vi "AIT 664 RT Driver VI.vi"(7 "Operation":T1, 11 "Device Reference in":T2 format="%.0x") -> (0 "Error Code":i32)   [LabVIEW 2014, in "AIT 664 Custom Device.lvlib"]
uses:
  AIT 664 Custom Device.lvlib
  <vilib>/NI Veristand/Custom Device API/Custom Device Item Ref.ctl
  <vilib>/NI Veristand/Custom Device API/Hardware Interface Driver VI Operation.ctl
  RT Controls/AIT 664  - RT Data.ctl
  RT Controls/AIT 664 - RT Hardware Channel.ctl
  RT Controls/AIT 664 - RT Message Settings.ctl
  <vilib>/NI Veristand/Custom Device API/Block Data Reference.ctl
  <vilib>/NI Veristand/Custom Device API/Data Reference.ctl
  RT Controls/AIT 664 - Driver Data.ctl
  Controls and Global/Start Bit.ctl
  Controls and Global/Number of Bits.ctl
  <userlib>/ARINC 664/AIT 664 Controls/General/Message Port.ctl
  <userlib>/ARINC 664/AIT 664 Controls/General/Direction.ctl
  <userlib>/ARINC 664/AIT 664 Controls/General/Message Port Type.ctl
  System Explorer/Controls/664 - Sampling Type.ctl
  RT Controls/Status Channels Config.ctl
  RT Controls/FIFO.ctl
  RT Controls/Label Transfer Config.ctl
  RT Controls/Async Loop Control Enum.ctl
  RT Controls/ReadWrite Selector.ctl
  SubVIs/Data Ref FGV.vi
  <vilib>/NI Veristand/Custom Device API/NI VeriStand - Set Channel Value by Data Reference.vi
  SubVIs/Error/Push Error if Different.vi
  <instrlib>/AIT 664/Private/AIT 664 Configure/Rx/Close/AIT 664 Rx Close Message Port (ComUdp).vi
  <instrlib>/AIT 664/Private/AIT 664 Configure/Tx/Close/AIT 664 Tx Close Message Port (ComUdp).vi
  <vilib>/NI Veristand/Custom Device API/Global Data Refs.vi
  SubVIs/Init/AIT 664 - Get Index and Length.vi
  SubVIs/Init/AIT 664 - Parse Channels.vi
  <vilib>/NI Veristand/Custom Device API/Custom Device API.lvlib
  <userlib>/ARINC 664/AIT 664 API.lvlib
  <instrlib>/AIT 664/AIT 664.lvlib
  <vilib>/NI Veristand/Custom Device Tools/Custom Device Utility Library/Custom Device Utility Library.lvlib
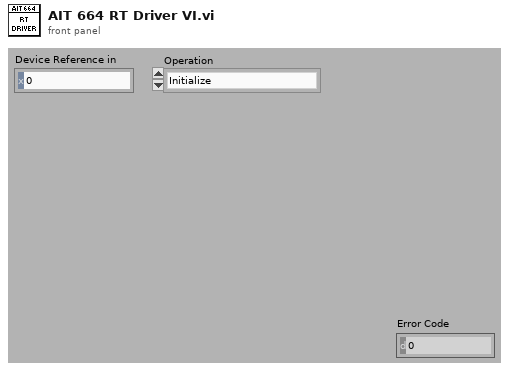
[diagram p1: front panel]
types:
  T1 = typedef "Custom Device API.lvlib/Hardware Interface Driver VI Operation.ctl" = enum16{"Initialize", "Start", "Read Data from HW", "Write Data to HW", "Close"}
  T2 = typedef "Custom Device API.lvlib/Custom Device Item Ref.ctl" = u64
  T3 = typedef "AIT 664 Custom Device.lvlib/AIT 664  - RT Data.ctl" = cluster{"Hardware Input Rx Channels":T4[], "Hardware Output Tx Channels":T4[], "Start":refnum<notifier>, "Error Publish Queue":refnum<queue>, "Error Queues":refnum<queue>[], "Status Config":T15, "FIFOs":T16, "VI References":refnum<vi>[], "Label Transfer Config":T17, "End System Handle ":u64}
  T4 = typedef "AIT 664 Custom Device.lvlib/AIT 664 - RT Hardware Channel.ctl" = cluster{"Channel Number":u16, "Message Name":string, "Message Settings":T5, "Tx Com Udp Port":T11, "Rx Com Udp Port":T11, "Rate (ms)":u32, "Sampling Type":T14}
  T5 = typedef "AIT 664 Custom Device.lvlib/AIT 664 - RT Message Settings.ctl" = cluster{"Name":string, "xmlName":string, "Tx-Rx_T-Tx":bool, "RT_Address":u8, "RT_SA_Address":u8, "Block Data Refs":T6[], "Values Array":dbl[], "Length":i32, "Words":i32, "FIFO Index":i32, "RX Word":u32, "IterationOffset":i32, "Default Msg Data":u8[], "Driver Data":T8, "Status Data":u32[], "Queue Transmit Channel":T2, "Transmit Channel Data Reference":T7}
  T6 = typedef "Custom Device API.lvlib/Block Data Reference.ctl" = cluster{"Data Reference":T7, "Offset":i32, "Length":i32}
  T7 = typedef "Custom Device API.lvlib/Data Reference.ctl" = i32
  T8 = typedef "AIT 664 Custom Device.lvlib/AIT 664 - Driver Data.ctl" = cluster{"First Word":T9[], "Start Bit":T9[], "Num Bits":T10[], "Decimation":i32, "IterationOffset":i32, "Signed?":bool[], "ScaleFac":dbl[], "ScaleOffset":dbl[]}
  T9 = typedef "AIT 664 Custom Device.lvlib/Start Bit.ctl" = i32
  T10 = typedef "AIT 664 Custom Device.lvlib/Number of Bits.ctl" = i32
  T11 = typedef "AIT 664 API.lvlib/Message Port.ctl" = cluster{"Direction":T12, "Type":T13, "Handle":u64}
  T12 = typedef "AIT 664 API.lvlib/Direction.ctl" = enum16{"DIRECTION_NONE", "DIRECTION_TX", "DIRECTION_RX"}
  T13 = typedef "AIT 664 API.lvlib/Message Port Type.ctl" = enum16{"PORT_TYPE_NONE", "COM_UDP", "SAP_UDP", "SAP_IP", "SAP_MAC", "COTS_MAC", "COTS_MAC_RAW"}
  T14 = typedef "AIT 664 Custom Device.lvlib/664 - Sampling Type.ctl" = enum16{"Com Udp", "Com Udp Queuing", "Sap Udp", "Sap Ip", "Sap Mac", "Unknown"}
  T15 = typedef "AIT 664 Custom Device.lvlib/Status Channels Config.ctl" = cluster{"Error Data Reference":T7, "Hardware In Count Reference":T7, "Hardware In Count Index":i32, "Hardware Out Count Reference":T7, "Hardware Out Count Index":i32, "Hardware In Dur Reference":T7, "Hardware In Dur Index":i32, "Hardware Out Dur Reference":T7, "Hardware Out Dur Index":i32}
  T16 = typedef "AIT 664 Custom Device.lvlib/FIFO.ctl" = cluster{"Hardware In FIFOs":refnum<k33>[], "Hardware Out FIFOs":refnum<k33>[], "Hardware In Buffer":dbl[], "Hardware Out Buffer":dbl[], "Empty Hardware In FIFOs":bool[], "Hardware In Buffer Indices":i32[], "Hardware Out Buffer Indices":i32[], "Hardware In Buffer Lengths":i32[], "Hardware Out Buffer Lengths":i32[]}
  T17 = typedef "AIT 664 Custom Device.lvlib/Label Transfer Config.ctl" = cluster{"Block Data Refs":T6[], "Values Array":dbl[]}
  T18 = typedef "AIT 664 Custom Device.lvlib/Async Loop Control Enum.ctl" = enum16{"Launch", "Start", "Stop"}
  T19 = typedef "AIT 664 Custom Device.lvlib/ReadWrite Selector.ctl" = enum16{"Inline Read", "Inline Write", "Async HWIn", "Async HWOut"}
  T20 = typedef "AIT 664 Custom Device.lvlib/FIFO Index Queues.ctl" = cluster{"Hardware Input Queue":refnum<queue>, "Hardware Output Queue":refnum<queue>}
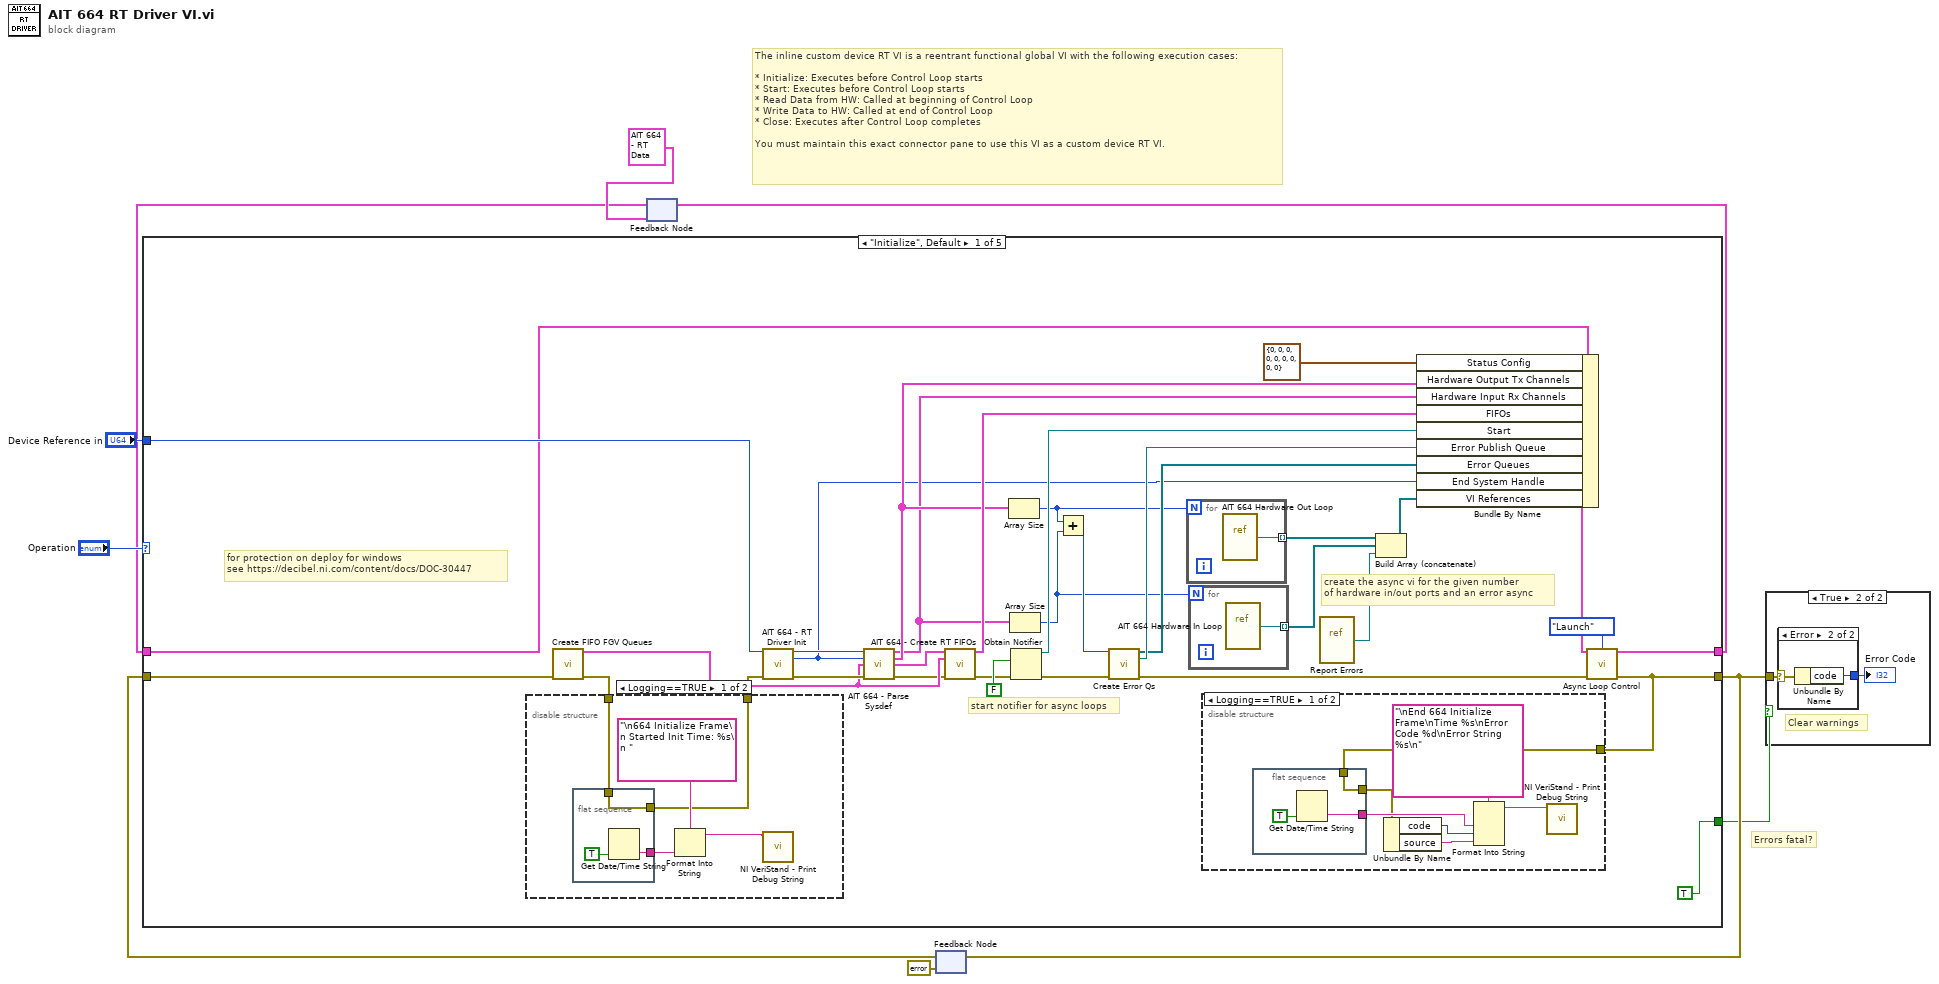
[diagram p0: block diagram]
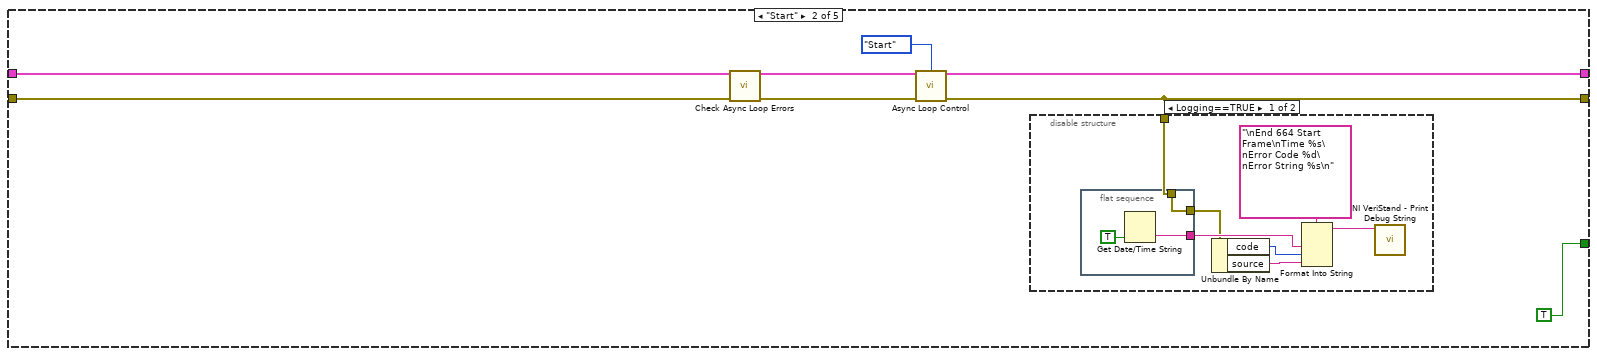
[diagram p6: hidden frame]
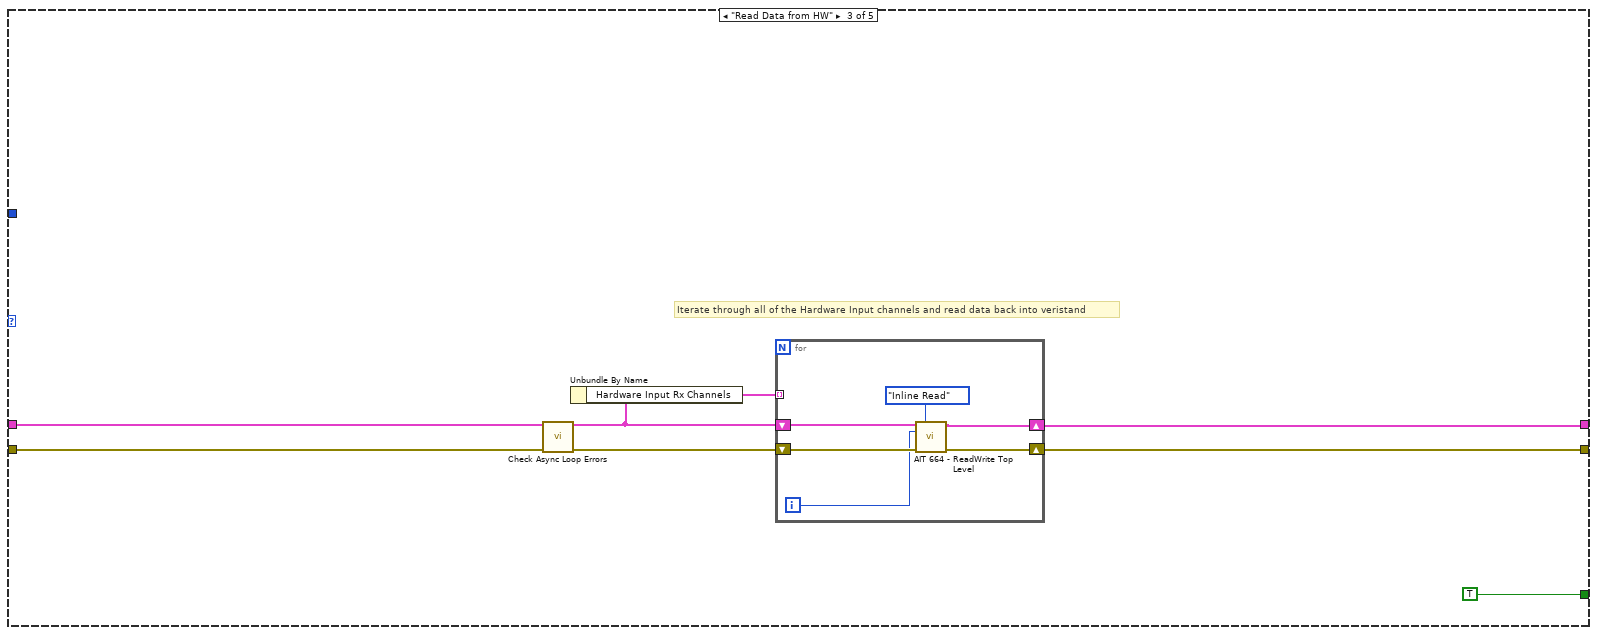
[diagram p8: hidden frame]
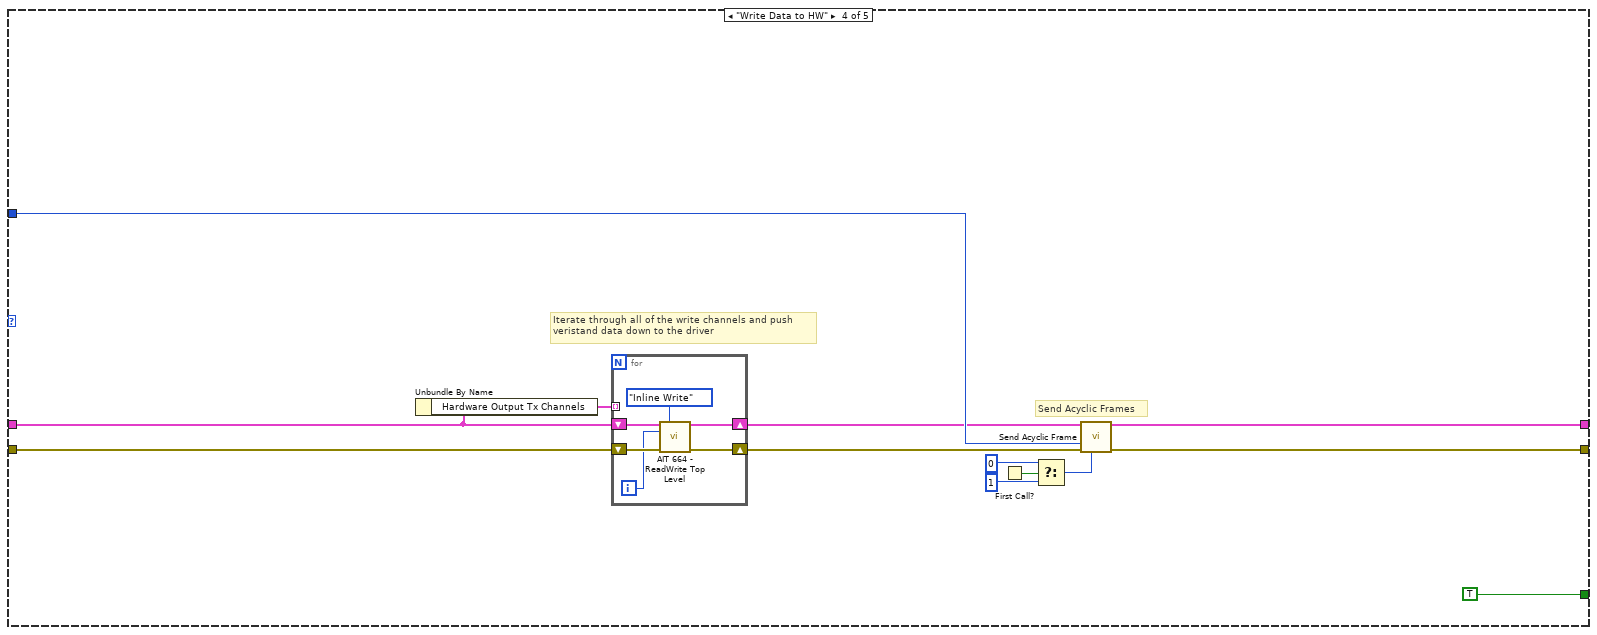
[diagram p9: hidden frame]
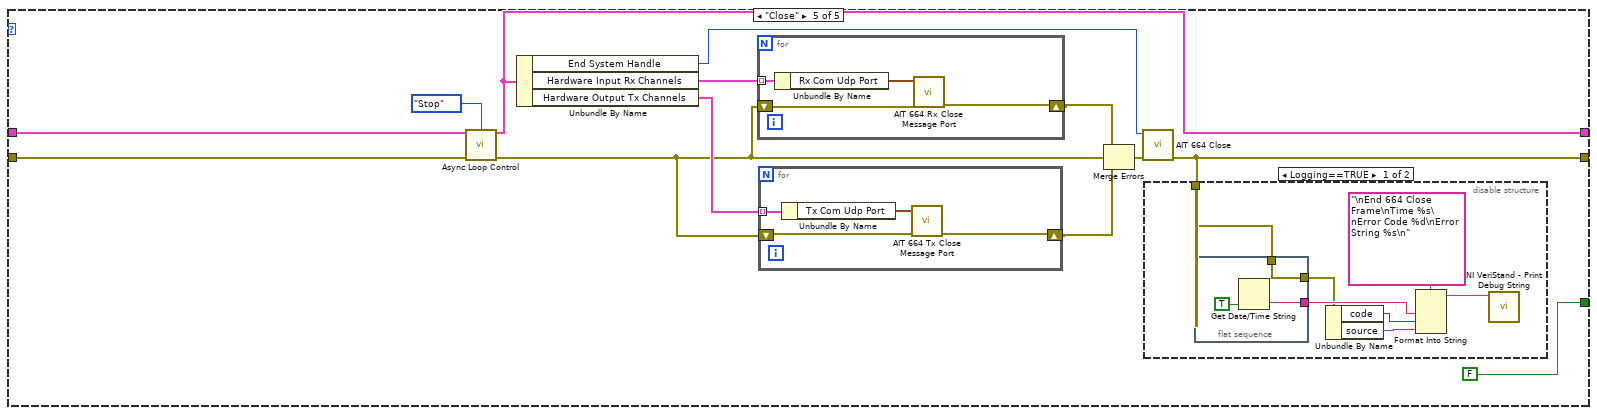
[diagram p10: hidden frame]
diagram:
  # "Errors fatal?"
  # "The inline custom device RT VI is a reentrant functional global VI with the following execution cases:\n\n* Initialize: Executes before Control Loop starts\n* Start: Executes before Control Loop starts\n* Read Data from HW: Called at beginning of Control Loop\n* Write Data to HW: Called at end of Control Loop\n* Close: Executes after Control Loop completes\n\nYou must maintain this exact connector pane to use this VI as a custom device RT VI."
  n1 = feedback #1(T3 {"Hardware Input Rx Channels"=[], "Hardware Output Tx Channels"=[], "Start"=refnum, "Error Publish Queue"=refnum, "Error Queues"=[], "Status Config"={"Error Data Reference"=0, "Hardware In Count Reference"=0, "Hardware In Count Index"=0, "Hardware Out Count Reference"=0, "Hardware Out Count Index"=0, "Hardware In Dur Reference"=0, "Hardware In Dur Index"=0, "Hardware Out Dur Reference"=0, "Hardware Out Dur Index"=0}, "FIFOs"={"Hardware In FIFOs"=[], "Hardware Out FIFOs"=[], "Hardware In Buffer"=[], "Hardware Out Buffer"=[], "Empty Hardware In FIFOs"=[], "Hardware In Buffer Indices"=[], "Hardware Out Buffer Indices"=[], "Hardware In Buffer Lengths"=[], "Hardware Out Buffer Lengths"=[]}, "VI References"=[], "Label Transfer Config"={"Block Data Refs"=[], "Values Array"=[]}, "End System Handle "=0} ("RT Data")) -> (w1:T3)
  n2 = feedback #2(errorcluster {"status"=FALSE, "code"=0, "source"=""} ("error out")) -> (w6:errorcluster)
  n3 = case shown="\"Initialize\", Default" "Operation" {
    tunnel: w1 -> [w35 w70 w88 w103 w126]
    tunnel: "Device Reference in" -> [w39 _ _ w106 _]
    tunnel: [w10 w65 w86 w107 w116] -> w7
    tunnel: w6 -> [w42 w72 w90 w109 w128]
    tunnel: [TRUE TRUE TRUE TRUE FALSE] -> w5
    tunnel: [w36 w69 w85 w97 w125] -> w2
    frame "Initialize", Default {
      # "for protection on deploy for windows\nsee https://decibel.ni.com/content/docs/DOC-30447"
      # "create the async vi for the given number\nof hardware in/out ports and an error async"
      # "start notifier for async loops"
      n4 = call "Create FIFO FGV Queues.vi"("error in (no error)"=w42) -> ("FIFO Index Queues"=w14:T20, "error out"=w40:errorcluster)  [unwired: 13 in]
      n5 = disable-structure shown="Logging==TRUE" {
        disable-tunnel: w40 -> [w46 w52]
        disable-tunnel: [w44 w52] -> w16
        frame condition #0 (active) {
          n6 = flat-sequence {
            tunnel: [w51] -> w47
            tunnel: w46 -> [w49]
            tunnel: [w49] -> w44
            frame #0 {
              n7 = Get Date/Time String(want seconds? (F)=TRUE) -> (time string=w51:string)  [unwired: 2 in, 1 out]
            }
          }
          n8 = Format Into String(format string="\n664 Initialize Frame\n Started Init Time: %s\n ", w47) -> (resulting string=w45:string)  [unwired: 2 in, 1 out]
          n9 = call <vilib>:"NI VeriStand - Print Debug String.vi"("Message"=w45) -> ()  [unwired: 10 in, 1 out]
        }
        frame condition #1 {
        }
      }
      n10 = call "AIT 664 - RT Driver Init.vi"("Device Reference in"=w39, "error in"=w16) -> ("Device Reference out"=w38:T2, "End System Handle out"=w13:u64, "error out"=w37:errorcluster)  [unwired: 11 in]
      n11 = call "AIT 664 - Parse Sysdef.vi"("Device Reference in"=w38, "End System Handle in"=w13, "FIFO Index Queues"=w14, "error in (no error)"=w37) -> ("Hardware Input - Rx Section Data"=w15:T4[], "Hardware Output - Tx Section Data"=w17:T4[], "output cluster"=w34:T16, "error out"=w12:errorcluster)  [unwired: 8 in]
      n12 = call "AIT 664 - Create RT FIFOs.vi"("input cluster"=w34, "FIFO Index Queues"=w14, "error in (no error)"=w12) -> ("output cluster"=w31:T16, "error out"=w33:errorcluster)  [unwired: 11 in]
      n13 = Array Size(array=w17) -> (size(s)=w18:i32)
      n14 = Array Size(array=w15) -> (size(s)=w19:i32)
      n15 = Obtain Notifier(notification data type=FALSE, error in (no error)=w33) -> (notifier out=w32:refnum<notifier>, error out=w29:errorcluster)  [unwired: 2 in, 1 out]
      n16 = Add(x=w18, y=w19) -> (x+y=w28:i32)
      n17 = call "Create Error Qs.vi"("Number of Error Queues to Create"=w28, "error in (no error)"=w29) -> ("Error Queues"=w26:refnum<queue>[], "Error Publishing Queue"=w27:refnum<queue>, "error out"=w11:errorcluster)  [unwired: 11 in]
      n18 = for {
        N: w18 -> [_]
        tunnel: [w63] -> w25 mode=indexing
        n19 = vi-ref "AIT 664 Hardware Out Loop.vi"() -> (w63:refnum<vi>)
      }
      n20 = for {
        N: w19 -> [_]
        tunnel: [w64] -> w24 mode=indexing
        n21 = vi-ref "AIT 664 Hardware In Loop.vi"() -> (w64:refnum<vi>)
      }
      n22 = vi-ref "Report Errors.vi"() -> (w20:refnum<vi>)
      n23 = Build Array (concatenate)(w25, w24, w20) -> (w23:refnum<vi>[])
      n24 = Bundle By Name(cluster=w35, "Status Config"=T15 {"Error Data Reference"=0, "Hardware In Count Reference"=0, "Hardware In Count Index"=0, "Hardware Out Count Reference"=0, "Hardware Out Count Index"=0, "Hardware In Dur Reference"=0, "Hardware In Dur Index"=0, "Hardware Out Dur Reference"=0, "Hardware Out Dur Index"=0}, "Hardware Output Tx Channels"=w17, "Hardware Input Rx Channels"=w15, "FIFOs"=w31, "Start"=w32, "Error Publish Queue"=w27, "Error Queues"=w26, "End System Handle"=w13, "VI References"=w23) -> (w22:T3)
      n25 = call "Async Loop Control.vi"("RT Data In"=w22, "Action"=Async_Loop_Control_Enum."Launch", "error in (no error)"=w11) -> ("RT Data Out"=w36:T3, "error out"=w10:errorcluster)  [unwired: 11 in]
      n26 = disable-structure shown="Logging==TRUE" {
        disable-tunnel: w10 -> [w55 _]
        frame condition #0 (active) {
          n27 = flat-sequence {
            tunnel: [w62] -> w58
            tunnel: w55 -> [w60]
            tunnel: [w60] -> w56
            frame #0 {
              n28 = Get Date/Time String(want seconds? (F)=TRUE) -> (time string=w62:string)  [unwired: 2 in, 1 out]
            }
          }
          n29 = Unbundle By Name(w56) -> ("code"=w57:i32, "source"=w59:string)
          n30 = Format Into String(format string="\nEnd 664 Initialize Frame\nTime %s\nError Code %d\nError String %s\n", w58, w57, w59) -> (resulting string=w54:string)  [unwired: 2 in, 1 out]
          n31 = call <vilib>:"NI VeriStand - Print Debug String.vi"("Message"=w54) -> ()  [unwired: 10 in, 1 out]
        }
        frame condition #1 {
        }
      }
    }
    frame "Start" {
      n32 = call "Check Async Loop Errors.vi"("RT Data in"=w70, "error in (no error)"=w72) -> ("RT Data Out"=w66:T3, "error out"=w67:errorcluster)  [unwired: 12 in]
      n33 = call "Async Loop Control.vi"("RT Data In"=w66, "Action"=Async_Loop_Control_Enum."Start", "error in (no error)"=w67) -> ("RT Data Out"=w69:T3, "error out"=w65:errorcluster)  [unwired: 11 in]
      n34 = disable-structure shown="Logging==TRUE" {
        disable-tunnel: w65 -> [w75 _]
        frame condition #0 (active) {
          n35 = flat-sequence {
            tunnel: [w82] -> w78
            tunnel: w75 -> [w80]
            tunnel: [w80] -> w76
            frame #0 {
              n36 = Get Date/Time String(want seconds? (F)=TRUE) -> (time string=w82:string)  [unwired: 2 in, 1 out]
            }
          }
          n37 = Unbundle By Name(w76) -> ("code"=w77:i32, "source"=w79:string)
          n38 = Format Into String(format string="\nEnd 664 Start Frame\nTime %s\nError Code %d\nError String %s\n", w78, w77, w79) -> (resulting string=w74:string)  [unwired: 2 in, 1 out]
          n39 = call <vilib>:"NI VeriStand - Print Debug String.vi"("Message"=w74) -> ()  [unwired: 10 in, 1 out]
        }
        frame condition #1 {
        }
      }
    }
    frame "Read Data from HW" {
      # "Iterate through all of the Hardware Input channels and read data back into veristand"
      n40 = call "Check Async Loop Errors.vi"("RT Data in"=w88, "error in (no error)"=w90) -> ("RT Data Out"=w84:T3, "error out"=w87:errorcluster)  [unwired: 12 in]
      n41 = Unbundle By Name(w84) -> ("Hardware Input Rx Channels"=w83:T4[])
      n42 = for {
        tunnel: w83 -> [_] mode=indexing
        shift-right: [w94] -> w86
        shift-left: w87 -> [w96]
        shift-right: [w93] -> w85
        shift-left: w84 -> [w92]
        i -> [w91]
        n43 = call "AIT 664 - ReadWrite Top Level.vi"("RT Data in"=w92, "Mode"=ReadWrite_Selector."Inline Read", "Channel Index"=w91, "error in (no error)"=w96) -> ("RT Data out"=w93:T3, "error out"=w94:errorcluster)  [unwired: 10 in]
      }
    }
    frame "Write Data to HW" {
      # "Iterate through all of the write channels and push \nveristand data down to the driver"
      # "Send Acyclic Frames"
      n44 = Unbundle By Name(w103) -> ("Hardware Output Tx Channels"=w102:T4[])
      n45 = for {
        tunnel: w102 -> [_] mode=indexing
        shift-right: [w112] -> w104
        shift-left: w103 -> [w111]
        shift-right: [w113] -> w105
        shift-left: w109 -> [w115]
        i -> [w110]
        n46 = call "AIT 664 - ReadWrite Top Level.vi"("RT Data in"=w111, "Mode"=ReadWrite_Selector."Inline Write", "Channel Index"=w110, "error in (no error)"=w115) -> ("RT Data out"=w112:T3, "error out"=w113:errorcluster)  [unwired: 10 in]
      }
      n47 = First Call?() -> (First Call?: T/F=w101:bool)
      n48 = Select(t=0 ("Index"), s=w101, f=1 ("Index")) -> (s? t:f=w98:i32)
      n49 = call "Send Acyclic Frame.vi"("RT Data in"=w104, "Device Reference in"=w106, "error in (no error)"=w105, "Index"=w98) -> ("RT Data out"=w97:T3, "error out"=w107:errorcluster)  [unwired: 10 in]
    }
    frame "Close" {
      n50 = call "Async Loop Control.vi"("RT Data In"=w126, "Action"=Async_Loop_Control_Enum."Stop", "error in (no error)"=w128) -> ("RT Data Out"=w125:T3, "error out"=w118:errorcluster)  [unwired: 11 in]
      n51 = Unbundle By Name(w125) -> ("End System Handle"=w120:u64, "Hardware Input Rx Channels"=w123:T4[], "Hardware Output Tx Channels"=w122:T4[])
      n52 = for {
        tunnel: w123 -> [w146] mode=indexing
        shift-right: [w143] -> w119
        shift-left: w118 -> [w144]
        n53 = Unbundle By Name(w146) -> ("Rx Com Udp Port"=w145:T11)
        n54 = call-poly <instrlib>:"AIT 664 Rx Close Message Port.vi"("error in"=w144, "Rx Com Udp Port in"=w145) -> ("error out"=w143:errorcluster)  [unwired: 7 in]
      }
      n55 = for {
        tunnel: w122 -> [w142] mode=indexing
        shift-right: [w139] -> w117
        shift-left: w118 -> [w140]
        n56 = Unbundle By Name(w142) -> ("Tx Com Udp Port"=w141:T11)
        n57 = call-poly <instrlib>:"AIT 664 Tx Close Message Port.vi"("error in"=w140, "Tx Com Udp Port in"=w141) -> ("error out"=w139:errorcluster)  [unwired: 7 in]
      }
      n58 = Merge Errors(w119, w118, w117) -> (w121:errorcluster)
      n59 = call <instrlib>:"AIT 664 Close.vi"("error in"=w121, "End System Handle in"=w120) -> ("error out"=w116:errorcluster)  [unwired: 9 in]
      n60 = disable-structure shown="Logging==TRUE" {
        disable-tunnel: w116 -> [w131 _]
        frame condition #0 (active) {
          n61 = flat-sequence {
            tunnel: [w138] -> w134
            tunnel: w131 -> [w136]
            tunnel: [w136] -> w132
            frame #0 {
              n62 = Get Date/Time String(want seconds? (F)=TRUE) -> (time string=w138:string)  [unwired: 2 in, 1 out]
            }
          }
          n63 = Unbundle By Name(w132) -> ("code"=w133:i32, "source"=w135:string)
          n64 = Format Into String(format string="\nEnd 664 Close Frame\nTime %s\nError Code %d\nError String %s\n", w134, w133, w135) -> (resulting string=w130:string)  [unwired: 2 in, 1 out]
          n65 = call <vilib>:"NI VeriStand - Print Debug String.vi"("Message"=w130) -> ()  [unwired: 10 in, 1 out]
        }
        frame condition #1 {
        }
      }
    }
  }
  n66 = feedback-in #1(w2) -> ()
  n67 = feedback-in #2(w7) -> ()
  n68 = case shown="True" w5 {
    tunnel: w7 -> [_ w147]
    frame False {
    }
    frame True {
      # "Clear warnings"
      n69 = case shown="Error" w147 {
        selector: w147 -> [_ w150]
        tunnel: [_ w149] -> w148
        frame No Error {
        }
        frame Error {
          n70 = Unbundle By Name(w150) -> ("code"=w149:i32)
        }
      }
      "Error Code" <- w148
    }
  }
